vi "Dice Indicator with Led Display.vi"() -> ()   [LabVIEW 2020]
panel:
  out "6":bool[][](array[boolean])
  out "5":bool[][](array[boolean])
  out "4":bool[][](array[boolean])
  out "3":bool[][](array[boolean])
  out "2":bool[][](array[boolean])
  in  "number":u64
  in  "stop":bool
  out "1":bool[][](array[boolean])
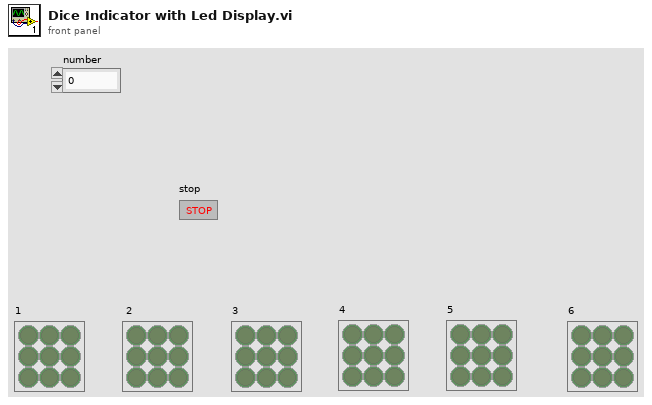
[diagram p1: front panel]
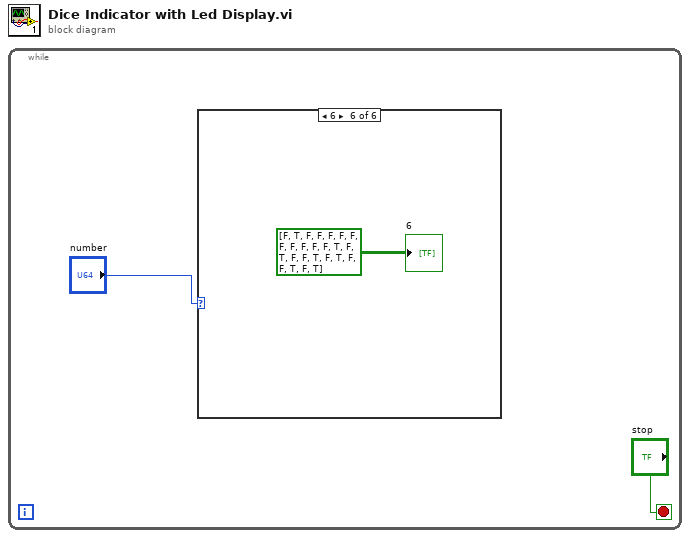
[diagram p0: block diagram]
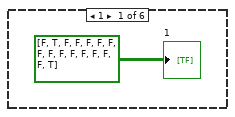
[diagram p2: hidden frame]
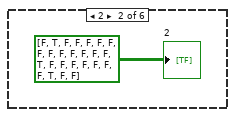
[diagram p3: hidden frame]
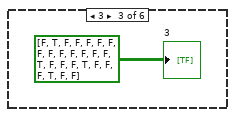
[diagram p4: hidden frame]
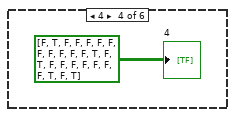
[diagram p5: hidden frame]
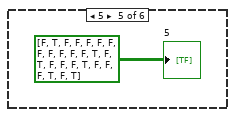
[diagram p6: hidden frame]
diagram:
  n1 = while {
    stop <- "stop" stop-if-true
    n2 = case shown="6" "number" {
      frame 1 {
        "1" <- bool[][] [[FALSE, TRUE, FALSE, FALSE], [FALSE, FALSE, FALSE, FALSE], [FALSE, FALSE, FALSE, FALSE], [FALSE, FALSE, FALSE, TRUE]] ("Array")
      }
      frame 2 {
        "2" <- bool[][] [[FALSE, TRUE, FALSE, FALSE, FALSE], [FALSE, FALSE, FALSE, FALSE, FALSE], [FALSE, FALSE, FALSE, FALSE, TRUE], [FALSE, FALSE, FALSE, FALSE, FALSE], [FALSE, FALSE, TRUE, FALSE, FALSE]] ("Array")
      }
      frame 3 {
        "3" <- bool[][] [[FALSE, TRUE, FALSE, FALSE, FALSE], [FALSE, FALSE, FALSE, FALSE, FALSE], [FALSE, FALSE, FALSE, FALSE, TRUE], [FALSE, FALSE, FALSE, TRUE, FALSE], [FALSE, FALSE, TRUE, FALSE, FALSE]] ("Array")
      }
      frame 4 {
        "4" <- bool[][] [[FALSE, TRUE, FALSE, FALSE, FALSE], [FALSE, FALSE, FALSE, FALSE, FALSE], [FALSE, FALSE, TRUE, FALSE, TRUE], [FALSE, FALSE, FALSE, FALSE, FALSE], [FALSE, FALSE, TRUE, FALSE, TRUE]] ("Array")
      }
      frame 5 {
        "5" <- bool[][] [[FALSE, TRUE, FALSE, FALSE, FALSE], [FALSE, FALSE, FALSE, FALSE, FALSE], [FALSE, FALSE, TRUE, FALSE, TRUE], [FALSE, FALSE, FALSE, TRUE, FALSE], [FALSE, FALSE, TRUE, FALSE, TRUE]] ("Array")
      }
      frame 6 {
        "6" <- bool[][] [[FALSE, TRUE, FALSE, FALSE, FALSE], [FALSE, FALSE, FALSE, FALSE, FALSE], [FALSE, FALSE, TRUE, FALSE, TRUE], [FALSE, FALSE, TRUE, FALSE, TRUE], [FALSE, FALSE, TRUE, FALSE, TRUE]] ("Array")
      }
    }
  }
